vi "Get Blocksize.vi"(8 "error in":errorcluster, 11 "Block Upload Initiate in":refnum<class "Block Upload Initiate Transfer.lvclass">) -> (0 "error out":errorcluster, 2 "Blocksize":u8=16, 3 "Block Upload Initiate out":refnum<class "Block Upload Initiate Transfer.lvclass">)   [LabVIEW 2020, in "CANopen.lvlib" / "SDO Manager.lvlib" / "Block Upload Initiate Transfer.lvclass"]
uses:
  Block Upload Initiate Transfer.lvclass
  Block Upload Initiate Transfer.lvclass/Block Upload Initiate Transfer.ctl
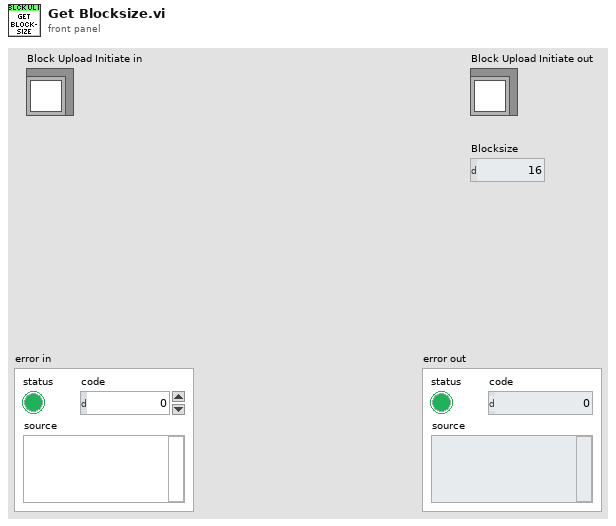
[diagram p1: front panel]
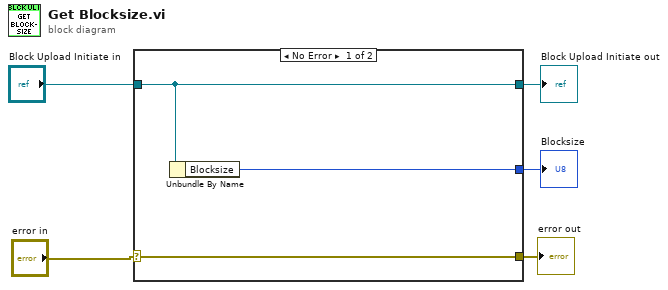
[diagram p0: block diagram]
diagram:
  n1 = case shown="No Error" "error in" {
    selector: "error in" -> [w8 w9]
    tunnel: [w8 w9] -> w2
    tunnel: [w7 w10] -> w4
    tunnel: "Block Upload Initiate in" -> [w7 w10]
    tunnel: [w6 _] -> w1
    frame No Error {
      n2 = Unbundle By Name(w7) -> ("Blocksize"=w6:u8)
    }
    frame Error {
    }
  }
  "error out" <- w2
  "Block Upload Initiate out" <- w4
  "Blocksize" <- w1
